vi "Curtin1_FavLists.vi"(6 "Task":enum16{"Save", "Read", "List", "Delete"}(ring), 8 "Default":string="favorites", 9 "List Name":string="favorites", 10 "description in":string, 11 "Files":T1[](array[typedef])) -> (1 "String":string, 2 "description out":string, 3 "Lists":string[](array[string]), 5 "Files Out":T1[](array[typedef]))   [LabVIEW 2022 SP3]
uses:
  Curtin1_Label.ctl
panel:
  out "error out":errorcluster
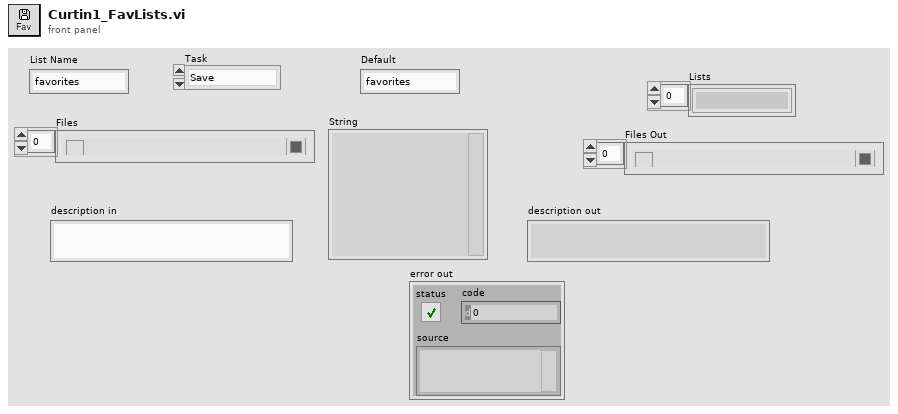
[diagram p1: front panel]
types:
  T1 = typedef "Curtin1_Label.ctl" = cluster{"Show?":bool, "Name":string, "Color":u32, "Path":path, "Show Notes":bool}
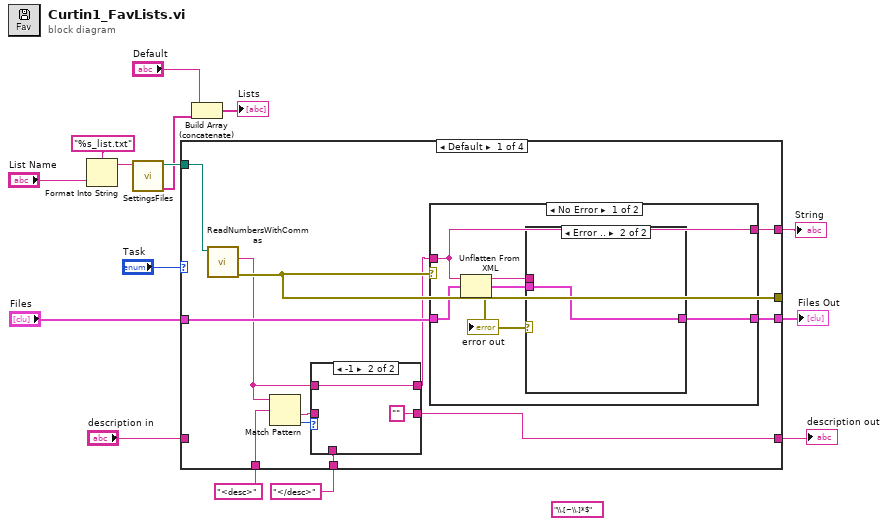
[diagram p0: block diagram]
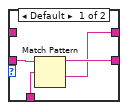
[diagram p2: hidden frame]
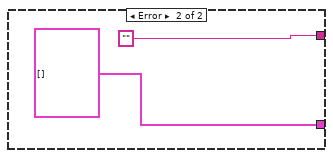
[diagram p4: hidden frame]
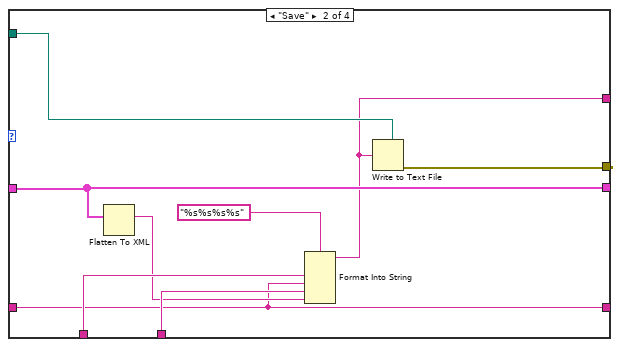
[diagram p5: hidden frame]
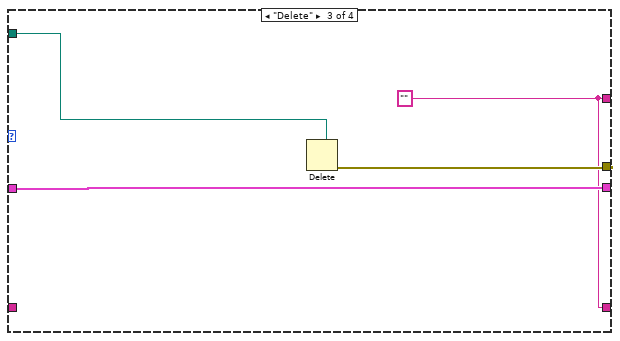
[diagram p6: hidden frame]
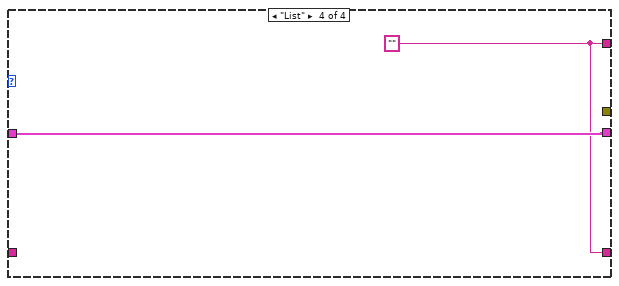
[diagram p7: hidden frame]
diagram:
  (unwired) "\\.[~\\.]*$" ("regular expression")
  n1 = Format Into String(format string="%s_list.txt" ("name or relative path"), "List Name") -> (resulting string=w4:string)  [unwired: 2 in, 1 out]
  n2 = call "SettingsFiles.vi"("settings file name"=w4) -> ("filenames"=w1:string[], "file path"=w3:path)  [unwired: 9 in]
  n3 = case shown="Default" "Task" {
    tunnel: "Files" -> [w26 w50 w54 w57]
    tunnel: [w24 w51 w55 _] -> _
    tunnel: [w27 w50 w54 w57] -> w10
    tunnel: [w25 w47 w52 w56] -> w13
    tunnel: w3 -> [w17 w49 w53 _]
    tunnel: [w18 w43 w52 w56] -> w8
    tunnel: "description in" -> [_ w43 _ _]
    tunnel: "<desc>" ("regular expression") -> [w23 w46 _ _]
    tunnel: "</desc>" ("regular expression") -> [w19 w45 _ _]
    frame Default {
      n4 = call "ReadNumbersWithCommas.vi"("file (use dialog)"=w17) -> ("error out"=w24:errorcluster, "text"=w21:string)  [unwired: 7 in, 2 out]
      n5 = Match Pattern(string=w21, regular expression=w23) -> (after substring=w20:string, offset past match=w22:i32)  [unwired: 1 in, 2 out]
      n6 = case shown="-1" w22 {
        tunnel: [w28 w33] -> w16
        tunnel: w21 -> [_ w33]
        tunnel: w20 -> [w31 _]
        tunnel: w19 -> [w30 _]
        tunnel: [w29 "" ("text")] -> w18
        frame Default {
          n7 = Match Pattern(string=w31, regular expression=w30) -> (before substring=w29:string, after substring=w28:string)  [unwired: 1 in, 2 out]
        }
        frame -1 {
        }
      }
      n8 = case shown="No Error" w24 {
        tunnel: [w35 T1[] [] ("Files")] -> w27
        tunnel: w16 -> [w36 _]
        tunnel: w26 -> [w38 _]
        tunnel: [w36 ""] -> w25
        frame No Error {
          n9 = Unflatten From XML(xml string=w36, type=w38) -> (value=w34:T1[], error out=w37:errorcluster)  [unwired: 1 in]
          "error out" <- w37
          n10 = case shown="Error .." w37 {
            tunnel: w36 -> [_ _]
            tunnel: [w39 w40] -> w35
            tunnel: w34 -> [w39 w40]
            frame No Error {
            }
            frame Error {
            }
          }
        }
        frame Error {
        }
      }
    }
    frame "Save" {
      n11 = Flatten To XML(6:w50) -> (2:w44:string)
      n12 = Format Into String(format string="%s%s%s%s", w46, w43, w45, w44) -> (resulting string=w47:string)  [unwired: 2 in, 1 out]
      n13 = Write to Text File(file (use dialog)=w49, text=w47) -> (error out=w51:errorcluster)  [unwired: 2 in, 2 out]
    }
    frame "Delete" {
      w52 = "" ("spreadsheet string")
      n14 = Delete(path (use dialog)=w53) -> (error out=w55:errorcluster)  [unwired: 4 in, 2 out]
    }
    frame "List" {
      w56 = "" ("spreadsheet string")
    }
  }
  "String" <- w13
  "Files Out" <- w10
  "description out" <- w8
  n15 = Build Array (concatenate)("Default", w1) -> (→"Lists":string[])
